vi "GlobalFGVsubvi.vi"(8 "error in (no error)":errorcluster, 10 "Initial position":i32, 11 "Enum":enum16{"Process 2", "Process 1", "Init", "read"}(ring)) -> (0 "error out":errorcluster, 2 "New position":i32)   [LabVIEW 2017]
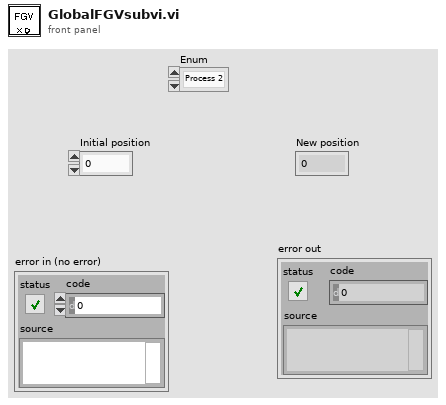
[diagram p1: front panel]
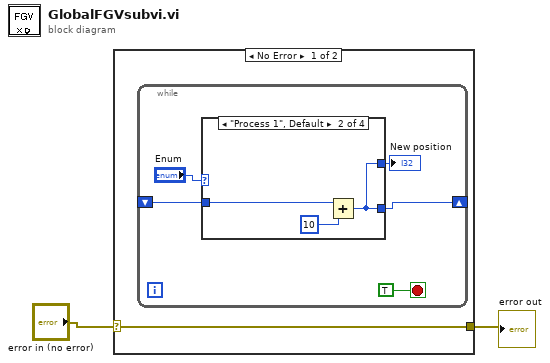
[diagram p0: block diagram]
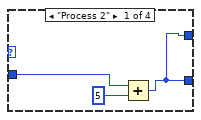
[diagram p2: hidden frame]
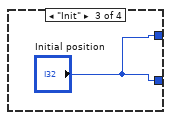
[diagram p3: hidden frame]
diagram:
  n1 = case shown="No Error" "error in (no error)" {
    selector: "error in (no error)" -> [w3 w17]
    tunnel: [w3 w17] -> w1
    frame No Error {
      n2 = while {
        shift-right: [w6] -> _
        shift-left: _ -> [w5]
        stop <- TRUE stop-if-true
        n3 = case shown="\"Process 1\", Default" "Enum" {
          tunnel: [w9 w12 "Initial position" w16] -> w6
          tunnel: w5 -> [w10 w13 _ w16]
          tunnel: [w9 w12 "Initial position" w16] -> w4
          frame "Process 2" {
            n4 = Add(x=w10, y=5) -> (x+y=w9:i32)
          }
          frame "Process 1", Default {
            n5 = Add(x=w13, y=10) -> (x+y=w12:i32)
          }
          frame "Init" {
          }
          frame "read" {
          }
        }
        "New position" <- w4
      }
    }
    frame Error {
    }
  }
  "error out" <- w1
